vi "Hoorizontal coords to select indent.vi"(8 "Coords.Horizontal":i32, 9 "Tree.Position:Left":i32, 10 "min allowed indent":i32, 11 "max allowed indent":i32) -> (3 "Coord Selected indent":i32)   [LabVIEW 2020, in "BetterDragAndDrop.lvlib" / "BetterTreeHandle.lvclass"]
uses:
  Classes/BetterTreeHandle/BetterTreeHandle.lvclass
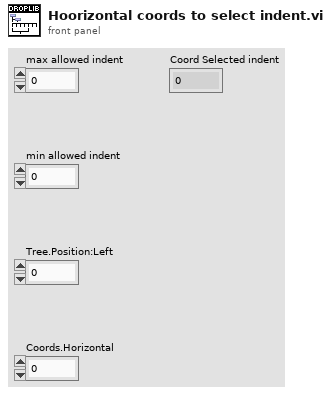
[diagram p1: front panel]
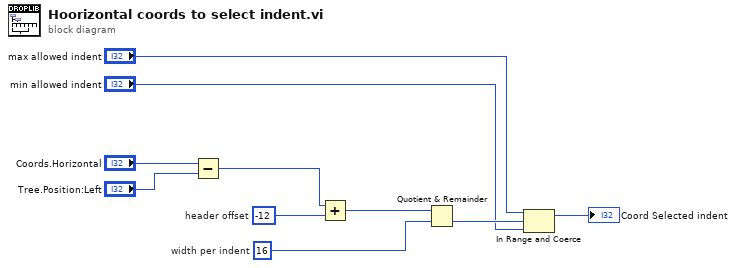
[diagram p0: block diagram]
diagram:
  w4 = -12  # header offset
  w8 = 16  # width per indent
  n1 = Subtract(x="Coords.Horizontal", y="Tree.Position:Left") -> (x-y=w5:i32)
  n2 = Add(x=w5, y=w4) -> (x+y=w3:i32)
  n3 = Quotient & Remainder(x=w3, y=w8) -> (floor(x/y)=w7:i32)  [unwired: 1 out]
  n4 = In Range and Coerce(upper limit="max allowed indent", x=w7, lower limit="min allowed indent") -> (coerced(x)=→"Coord Selected indent":i32)  [unwired: 1 out]
